vi "MH_DataInQueue.vi"(8 "error in (no error)":errorcluster, 10 "CountsHistos":T1, 11 "SinglePhotonInterferenceUI in":refnum<class "SinglePhotonInterferenceUI.lvclass">) -> (0 "error out":errorcluster, 3 "SinglePhotonInterferenceUI out":refnum<class "SinglePhotonInterferenceUI.lvclass">)   [LabVIEW 2023, in "SinglePhotonInterferenceUI.lvlib" / "SinglePhotonInterferenceUI.lvclass"]
uses:
  SinglePhotonInterferenceUI.lvclass
  CountsHistos.ctl
  typedefs/typedefs.lvlib
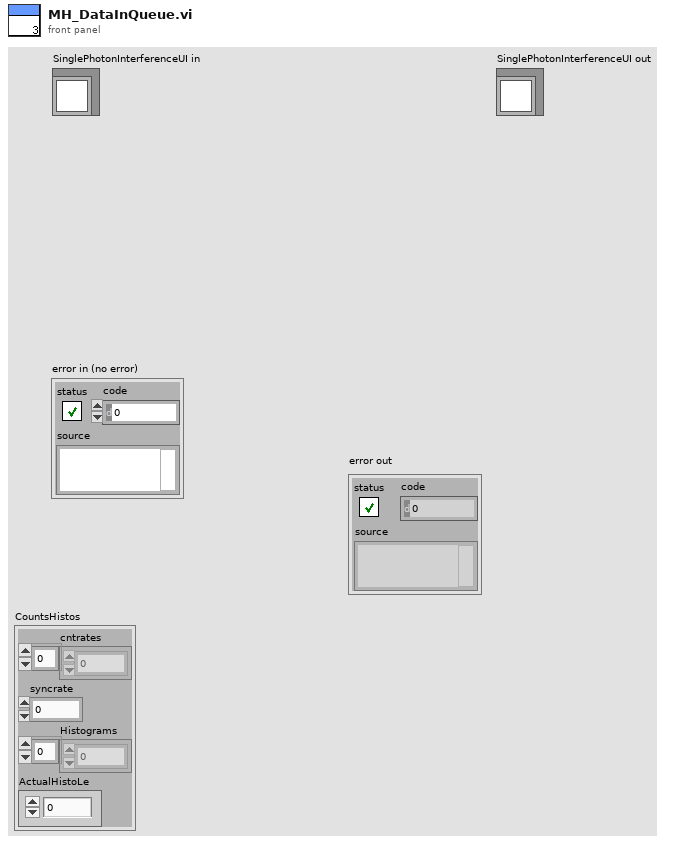
[diagram p1: front panel]
types:
  T1 = typedef "typedefs.lvlib/CountsHistos.ctl" = cluster{"cntrates":i32[], "syncrate":i32, "Histograms":u32[], "ActualHistoLe":i32}
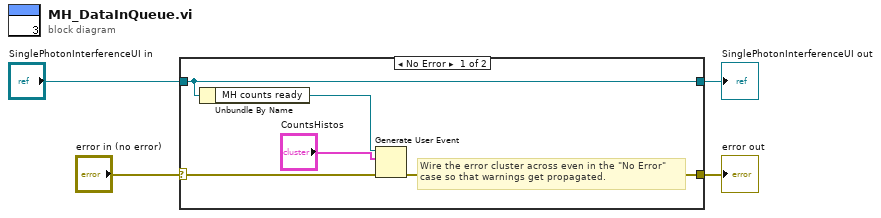
[diagram p0: block diagram]
diagram:
  n1 = case shown="No Error" "error in (no error)" {
    selector: "error in (no error)" -> [w6 w11]
    tunnel: [w5 w11] -> w1
    tunnel: [w9 w10] -> w3
    tunnel: "SinglePhotonInterferenceUI in" -> [w9 w10]
    frame No Error {
      # "Wire the error cluster across even in the \"No Error\"\ncase so that warnings get propagated."
      n2 = Unbundle By Name(w9) -> ("MH counts ready"=w8:refnum<user-event>)
      n3 = Generate User Event(user event=w8, event data cluster="CountsHistos", error in=w6) -> (error out=w5:errorcluster)  [unwired: 1 in, 1 out]
    }
    frame Error {
    }
  }
  "SinglePhotonInterferenceUI out" <- w3
  "error out" <- w1
